vi "RGB2Gray.vi"(9 "Blue":u8[][](array[numeric]), 10 "Green":u8[][](array[numeric]), 11 "Red":u8[][](array[numeric])) -> (3 "Array out":u8[][](array[numeric]))   [LabVIEW 2017, in "ImageAcquisitionLibrary.lvlib"]
uses:
  ImageAcquisitionLibrary.lvlib
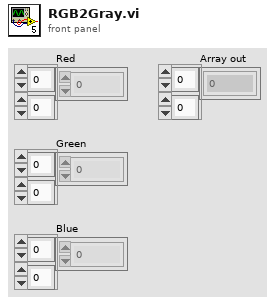
[diagram p1: front panel]
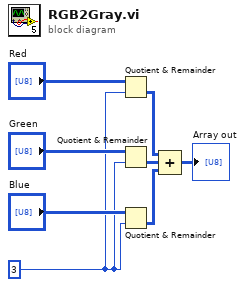
[diagram p0: block diagram]
diagram:
  w1 = u8 3
  n1 = Quotient & Remainder(x="Red", y=w1) -> (floor(x/y)=w5:u8[][])  [unwired: 1 out]
  n2 = Quotient & Remainder(x="Green", y=w1) -> (floor(x/y)=w6:u8[][])  [unwired: 1 out]
  n3 = Quotient & Remainder(x="Blue", y=w1) -> (floor(x/y)=w7:u8[][])  [unwired: 1 out]
  n4 = Compound Arithmetic op=ADD(w5, w6, w7) -> (→"Array out":u8[][])
